vi "InvertMotor.vi"(11 "Input":u16) -> (3 "Output":u16)   [LabVIEW 2013, in "ProcessorHelperFunctions.lvlib"]
uses:
  ProcessorHelperFunctions.lvlib
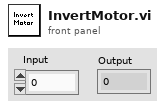
[diagram p1: front panel]
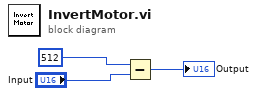
[diagram p0: block diagram]
diagram:
  n1 = Subtract(x=u16 512, y="Input") -> (x-y=→"Output":u16)
